vi "io_attr_write.vi"(7 "Attribute":T1={"Identifier"="", "Descriptive name"="", "Data Type"=enum."Integer 32", "Command"="", "Access"=2, "Range Table"="", "Read Callback"="", "Write Callback"="", "Range Callback"="", "Check Callback"="", "Rngtable Callback"="", "Coerce Callback"="", "Supported Models"="", "Instrument Options"="", "Repeated Capabilities"="", "Check Status Callback"="", "Index"=0, "Flag: OPC Wait"=FALSE, "Flag: Dont check status"=FALSE, "Flag: Cache Only"=FALSE} {"Access" items=["Read Only", "Write Only", "Read/Write"]}, 8 "error in":errorcluster, 10 "write buffer":string, 11 "VISA resource name":refnum<visa-resource-name>) -> (0 "error out":errorcluster, 3 "VISA resource name out":refnum<visa-resource-name>)   [LabVIEW 2014, in "rszvl_rsidr_core.lvlib"]
uses:
  rszvl_rsidr_core.lvlib
  type_Attribute.ctl
  type_Attribute_Data_Type.ctl
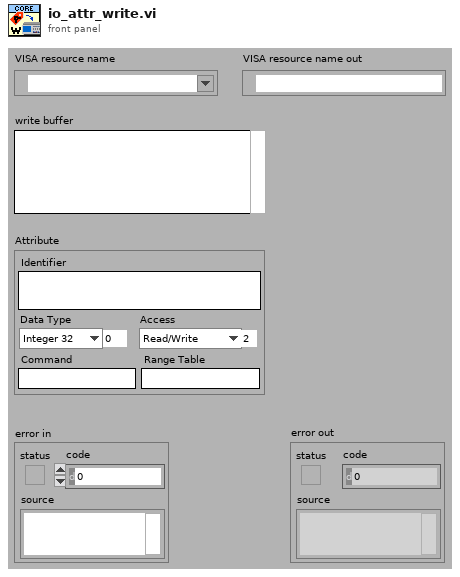
[diagram p1: front panel]
types:
  T1 = typedef "rszvl_rsidr_core.lvlib/type_Attribute.ctl" = cluster{"Identifier":string, "Descriptive name":string, "Data Type":T2, "Command":string, "Access":u16, "Range Table":string, "Read Callback":string, "Write Callback":string, "Range Callback":string, "Check Callback":string, "Rngtable Callback":string, "Coerce Callback":string, "Supported Models":string, "Instrument Options":string, "Repeated Capabilities":string, "Check Status Callback":string, "Index":i32, "Flag: OPC Wait":bool, "Flag: Dont check status":bool, "Flag: Cache Only":bool}
  T2 = typedef "rszvl_rsidr_core.lvlib/type_Attribute_Data_Type.ctl" = enum16{"Integer 32", "Double", "String", "Boolean", "None", "Integer 64"}
  T3 = typedef "rszvl_rsidr_core.lvlib/type_Session_Data.ctl" = cluster{"Instr type":string, "Instr type for err. msg.":string, "Installed Options":string[], "OPC Timeout":i32, "Query Instrument Status":bool, "Check Range":bool, "Check Options":bool, "Add LF to Write":bool, "Simulate":bool, "Logging":bool, "Logging params":variant, "Interface Type":enum16{"Unknown", "GPIB", "VXI", "GPIB_VXI", "ASRL", "PXI", "TCPIP", "USB", "SOCKET"}, "Fast Sweep":i32, "AdditionalFlags":i32, "WaitBeforeWrite":i32, "WaitBeforeRead":i32, "BinDataChunkSize":i64}
  T4 = enum16{"Unknown", "GPIB", "VXI", "GPIB_VXI", "ASRL", "PXI", "TCPIP", "USB", "SOCKET"}
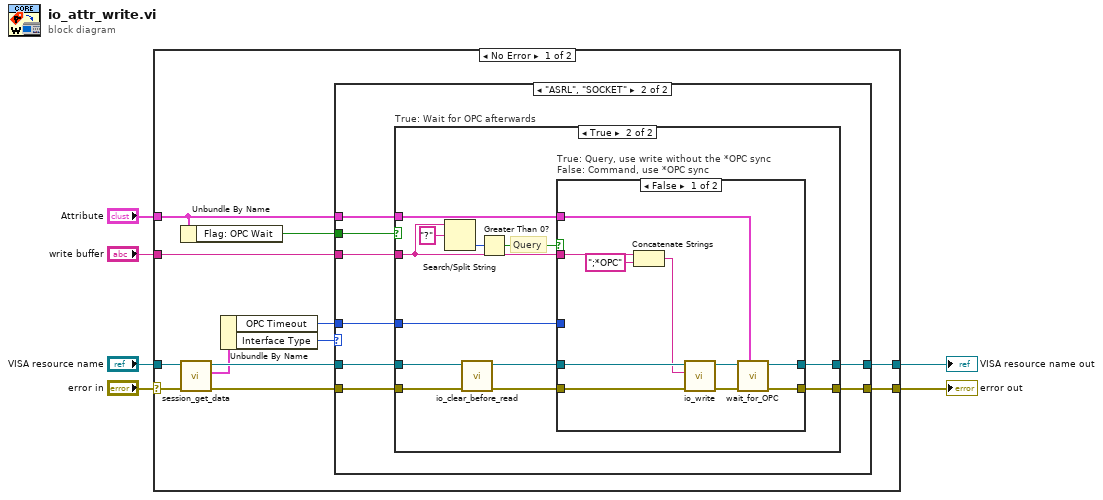
[diagram p0: block diagram]
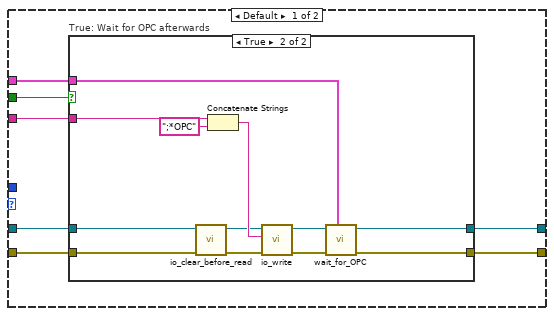
[diagram p2: hidden frame]
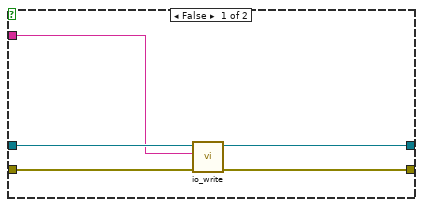
[diagram p3: hidden frame]
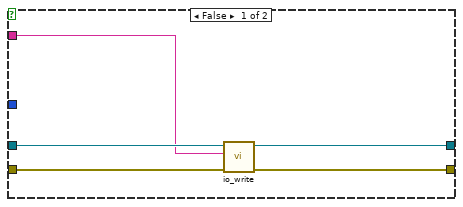
[diagram p4: hidden frame]
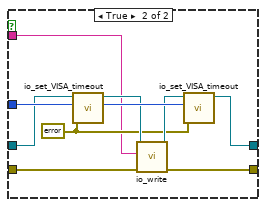
[diagram p5: hidden frame]
diagram:
  n1 = case shown="No Error" "error in" {
    selector: "error in" -> [w13 w89]
    tunnel: "VISA resource name" -> [w12 w88]
    tunnel: [w17 w89] -> w6
    tunnel: [w16 w88] -> w5
    tunnel: "Attribute" -> [w15 _]
    tunnel: "write buffer" -> [w14 _]
    frame No Error {
      n2 = Unbundle By Name(w15) -> ("Flag: OPC Wait"=w18:bool)
      n3 = call "session_get_data.vi"("error in"=w13, "VISA resource name"=w12) -> ("error out"=w11:errorcluster, "Session User Data out"=w9:T3, "VISA resource name out"=w10:refnum<visa-resource-name>)  [unwired: 7 in]
      n4 = Unbundle By Name(w9) -> ("OPC Timeout"=w7:i32, "Interface Type"=w8:T4)
      n5 = case shown="\"ASRL\", \"SOCKET\"" w8 {
        tunnel: w18 -> [w25 w50]
        tunnel: [w20 w45] -> w17
        tunnel: [w21 w46] -> w16
        tunnel: w11 -> [w24 w49]
        tunnel: w10 -> [w23 w48]
        tunnel: w15 -> [w19 w43]
        tunnel: w14 -> [w22 w47]
        tunnel: w7 -> [_ w44]
        frame Default {
          n6 = case "True: Wait for OPC afterwards" shown="True" w25 {
            tunnel: w22 -> [w26 w42]
            tunnel: w24 -> [w30 w40]
            tunnel: w23 -> [w29 w39]
            tunnel: [w28 w32] -> w20
            tunnel: [w27 w31] -> w21
            tunnel: w19 -> [_ w37]
            frame False {
              n7 = call "io_write.vi"("error in"=w30, "write buffer"=w26, "VISA resource name"=w29) -> ("error out"=w28:errorcluster, "VISA resource name out"=w27:refnum<visa-resource-name>)  [unwired: 7 in]
            }
            frame True {
              n8 = call "io_clear_before_read.vi"("error in"=w40, "VISA resource name"=w39) -> ("error out"=w36:errorcluster, "VISA resource name out"=w35:refnum<visa-resource-name>)  [unwired: 8 in]
              n9 = Concatenate Strings(w42, ";*OPC" ("string")) -> (w38:string)
              n10 = call "io_write.vi"("error in"=w36, "write buffer"=w38, "VISA resource name"=w35) -> ("error out"=w34:errorcluster, "VISA resource name out"=w33:refnum<visa-resource-name>)  [unwired: 7 in]
              n11 = call "wait_for_OPC.vi"("Attribute"=w37, "error in"=w34, "VISA resource name"=w33) -> ("error out"=w32:errorcluster, "VISA resource name out"=w31:refnum<visa-resource-name>)  [unwired: 7 in]
            }
          }
        }
        frame "ASRL", "SOCKET" {
          n12 = case "True: Wait for OPC afterwards" shown="True" w50 {
            tunnel: w47 -> [w51 w63]
            tunnel: w49 -> [w55 w66]
            tunnel: w48 -> [w54 w67]
            tunnel: [w53 w58] -> w45
            tunnel: [w52 w57] -> w46
            tunnel: w44 -> [_ w60]
            tunnel: w43 -> [_ w56]
            frame False {
              n13 = call "io_write.vi"("error in"=w55, "write buffer"=w51, "VISA resource name"=w54) -> ("error out"=w53:errorcluster, "VISA resource name out"=w52:refnum<visa-resource-name>)  [unwired: 7 in]
            }
            frame True {
              # "Query"
              n14 = Search/Split String(string=w63, search string/char (-)="?") -> (offset of match=w64:i32)  [unwired: 1 in, 2 out]
              n15 = call "io_clear_before_read.vi"("error in"=w66, "VISA resource name"=w67) -> ("error out"=w61:errorcluster, "VISA resource name out"=w59:refnum<visa-resource-name>)  [unwired: 8 in]
              n16 = Greater Than 0?(x=w64) -> (x > 0?=w62:bool)
              n17 = case "True: Query, use write without the *OPC sync\nFalse: Command, use *OPC sync" shown="False" w62 {
                tunnel: w63 -> [w76 w78]
                tunnel: w61 -> [w74 w84]
                tunnel: w60 -> [_ w87]
                tunnel: w59 -> [w73 w85]
                tunnel: [w70 w81] -> w58
                tunnel: [w69 w79] -> w57
                tunnel: w56 -> [w75 _]
                frame False {
                  n18 = Concatenate Strings(w76, ";*OPC" ("string")) -> (w68:string)
                  n19 = call "io_write.vi"("error in"=w74, "write buffer"=w68, "VISA resource name"=w73) -> ("error out"=w72:errorcluster, "VISA resource name out"=w71:refnum<visa-resource-name>)  [unwired: 7 in]
                  n20 = call "wait_for_OPC.vi"("Attribute"=w75, "error in"=w72, "VISA resource name"=w71) -> ("error out"=w70:errorcluster, "VISA resource name out"=w69:refnum<visa-resource-name>)  [unwired: 7 in]
                }
                frame True {
                  w80 = errorcluster {"status"=FALSE, "code"=0, "source"=""} ("error in")
                  n21 = call "io_set_VISA_timeout.vi"("error in"=w80, "VISA Timeout"=w87, "VISA resource name"=w85) -> ("Old VISA Timeout"=w86:u32, "VISA resource name out"=w83:refnum<visa-resource-name>)  [unwired: 6 in, 1 out]
                  n22 = call "io_write.vi"("error in"=w84, "write buffer"=w78, "VISA resource name"=w83) -> ("error out"=w81:errorcluster, "VISA resource name out"=w82:refnum<visa-resource-name>)  [unwired: 7 in]
                  n23 = call "io_set_VISA_timeout.vi"("error in"=w80, "VISA Timeout"=w86, "VISA resource name"=w82) -> ("VISA resource name out"=w79:refnum<visa-resource-name>)  [unwired: 6 in, 2 out]
                }
              }
            }
          }
        }
      }
    }
    frame Error {
    }
  }
  "VISA resource name out" <- w5
  "error out" <- w6
